vi "Convert Frequency.vi"(6 "Default (-999.00)":dbl=-999.0 format="%.2f", 7 "Units (Hz)":T1, 10 "String":string) -> (1 "Frequency":dbl format="%.10f", 2 "Units out":T1)   [LabVIEW 2015]
uses:
  Controls/Hz_KHz_MHz_GHz.ctl
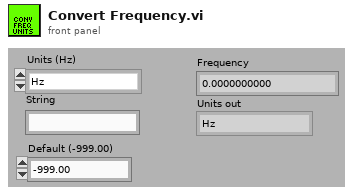
[diagram p1: front panel]
types:
  T1 = typedef "Hz_KHz_MHz_GHz.ctl" = enum16{"Hz", "KHz", "MHz", "GHz"}
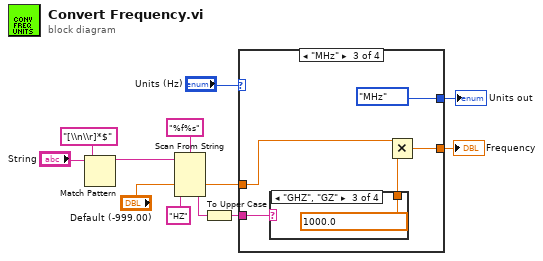
[diagram p0: block diagram]
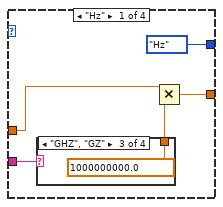
[diagram p2: hidden frame]
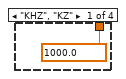
[diagram p3: hidden frame]
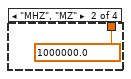
[diagram p4: hidden frame]
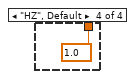
[diagram p5: hidden frame]
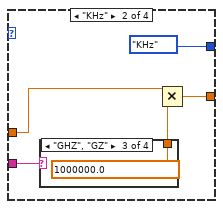
[diagram p6: hidden frame]
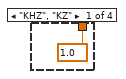
[diagram p7: hidden frame]
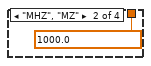
[diagram p8: hidden frame]
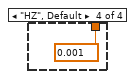
[diagram p9: hidden frame]
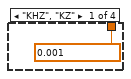
[diagram p10: hidden frame]
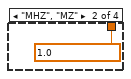
[diagram p11: hidden frame]
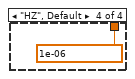
[diagram p12: hidden frame]
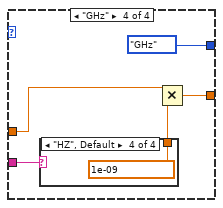
[diagram p13: hidden frame]
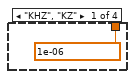
[diagram p14: hidden frame]
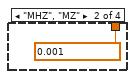
[diagram p15: hidden frame]
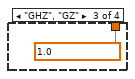
[diagram p16: hidden frame]
diagram:
  n1 = Match Pattern(string="String", regular expression="[\\n\\r]*$") -> (before substring=w4:string)  [unwired: 1 in, 3 out]
  n2 = Scan From String(format string="%f%s", input string=w4, default 1="Default (-999.00)", default 2="HZ" ("default value 2")) -> (output 1=w10:dbl, output 2=w3:string)  [unwired: 2 in, 3 out]
  n3 = To Upper Case(1:w3) -> (0:w2:string)
  n4 = case shown="\"MHz\"" "Units (Hz)" {
    tunnel: w10 -> [w16 w25 w34 w43]
    tunnel: w2 -> [w15 w26 w35 w44]
    tunnel: [w14 w23 w32 w41] -> w6
    tunnel: [Hz_KHz_MHz_GHz."Hz" ("Units out") Hz_KHz_MHz_GHz."KHz" ("Units out") Hz_KHz_MHz_GHz."MHz" ("Units out") Hz_KHz_MHz_GHz."GHz" ("Units out")] -> w5
    frame "Hz" {
      n5 = case shown="\"GHZ\", \"GZ\"" w15 {
        tunnel: [1000.0 1000000.0 1000000000.0 1.0] -> w17
        frame "KHZ", "KZ" {
        }
        frame "MHZ", "MZ" {
        }
        frame "GHZ", "GZ" {
        }
        frame "HZ", Default {
        }
      }
      n6 = Multiply(x=w16, y=w17) -> (x*y=w14:dbl)
    }
    frame "KHz" {
      n7 = case shown="\"GHZ\", \"GZ\"" w26 {
        tunnel: [1.0 1000.0 1000000.0 0.001] -> w24
        frame "KHZ", "KZ" {
        }
        frame "MHZ", "MZ" {
        }
        frame "GHZ", "GZ" {
        }
        frame "HZ", Default {
        }
      }
      n8 = Multiply(x=w25, y=w24) -> (x*y=w23:dbl)
    }
    frame "MHz" {
      n9 = case shown="\"GHZ\", \"GZ\"" w35 {
        tunnel: [0.001 1.0 1000.0 1e-06] -> w33
        frame "KHZ", "KZ" {
        }
        frame "MHZ", "MZ" {
        }
        frame "GHZ", "GZ" {
        }
        frame "HZ", Default {
        }
      }
      n10 = Multiply(x=w34, y=w33) -> (x*y=w32:dbl)
    }
    frame "GHz" {
      n11 = case shown="\"HZ\", Default" w44 {
        tunnel: [1e-06 0.001 1.0 1e-09] -> w42
        frame "KHZ", "KZ" {
        }
        frame "MHZ", "MZ" {
        }
        frame "GHZ", "GZ" {
        }
        frame "HZ", Default {
        }
      }
      n12 = Multiply(x=w43, y=w42) -> (x*y=w41:dbl)
    }
  }
  "Frequency" <- w6
  "Units out" <- w5
